vi "InitMiscellaneous.vi"   [LabVIEW 2020]
doc: "This VI initializes miscellaneous devices such as the compressor and any decorations."
uses:
  <vilib>/Rock Robotics/WPI/Compressor/WPI_CompressorFeedbackMode.ctl
  <vilib>/Rock Robotics/SystemInterfaces/DIO/FPGA_DIOPWMChannel.ctl
  GlobalMiscellaneous.vi
  <vilib>/Rock Robotics/WPI/Utilities/WPI_GetSetVariantRefNum.vi
types:
  T1 = typedef "FPGA_DIOPWMChannel.ctl" = enum8{"PWM 0", "PWM 1", "PWM 2", "PWM 3", "PWM 4", "PWM 5", "PWM 6", "PWM 7", "PWM 8", "PWM 9", "PWM MXP 0", "PWM MXP 1", "PWM MXP 2", "PWM MXP 3", "PWM MXP 4", "PWM MXP 5", "PWM MXP 6", "PWM MXP 7", "PWM MXP 8", "PWM MXP 9", "Invalid"}
  T2 = typedef "WPI_CompressorFeedbackMode.ctl" = enum16{"Analog Only", "Digital Only", "Hybrid"}
  T3 = cluster{"Feedback Sensor":T2, "Max Pressure (PSI)":dbl, "Min Pressure (PSI)":dbl}
  T4 = typedef "WPI_PWMDeviceRef.ctl" = cluster{"DeviceStatus":errorcluster, "PWM Channel":T1}
  T5 = typedef "WPI_CompressorDevRef.ctl" = cluster{"DevStatus":errorcluster, "Pneumatics Control Module":u8}
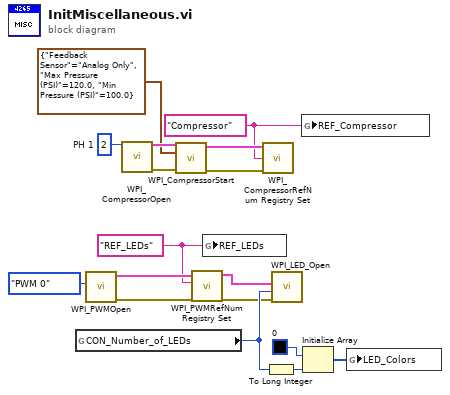
[diagram p0: block diagram]
diagram:
  w1 = "REF_LEDs" ("refnum name")
  w6 = "Compressor" ("refnum name")
  w14 = u8 2  # PH 1
  n1 = global read "GlobalMiscellaneous.vi" "CON_Number_of_LEDs"() -> (w7:u16)
  n2 = call <vilib>:"WPI_PWMOpen.vi"("PWM Channel"=FPGA_DIOPWMChannel."PWM 0") -> ("error out"=w5:errorcluster, "PWMDeviceRef"=w4:T4)  [unwired: 9 in]
  n3 = call <vilib>:"WPI_CompressorOpen.vi"("Pneumatics device (def)"=w14) -> ("CompressorDevRef"=w13:T5, "error out"=w10:errorcluster)  [unwired: 13 in]
  n4 = call <vilib>:"WPI_CompressorStart.vi"("error in (no error)"=w10, "Feedback Configuration"=T3 {"Feedback Sensor"=enum."Analog Only", "Max Pressure (PSI)"=120.0, "Min Pressure (PSI)"=100.0}, "CompressorDevRef"=w13) -> ("error out"=w9:errorcluster, "CompressorDevRef"=w11:T5)  [unwired: 7 in]
  n5 = call <vilib>:"WPI_PWMRefNum Registry Set.vi"("error in (no error)"=w5, "refnum name"=w1, "PWMDeviceRef"=w4) -> ("error out"=w2:errorcluster, "PWMDeviceRef"=w3:T4)  [unwired: 7 in]
  n6 = global write "GlobalMiscellaneous.vi" "REF_LEDs"(w1) -> ()
  n7 = call <vilib>:"WPI_CompressorRefNum Registry Set.vi"("error in (no error)"=w9, "refnum name"=w6, "CompressorDevRef"=w11) -> ()  [unwired: 7 in, 2 out]
  n8 = To Long Integer(number=w7) -> (32bit integer=w17:i32)
  n9 = call <vilib>:"WPI_LED_Open.vi"("error in"=w2, "String Length"=w7, "PWMDeviceRef"=w3) -> ()  [unwired: 8 in, 1 out]
  n10 = global write "GlobalMiscellaneous.vi" "REF_Compressor"(w6) -> ()
  n11 = Initialize Array(u32 0, w17) -> (w15:u32[])
  n12 = global write "GlobalMiscellaneous.vi" "LED_Colors"(w15) -> ()
